vi "CF_Read_Config.vi"(4 "error in (no error)":errorcluster, 7 "Config Refnum":T1) -> (0 "error out":errorcluster, 2 "All Found?":bool, 3 "refnum out":T1)   [LabVIEW 2015]
uses:
  <vilib>/Utility/config.llb/Config Data RefNum.ctl
  <vilib>/Utility/config.llb/Read Key (Double).vi
  GSP_CF_Global.vi
  <vilib>/Utility/config.llb/NI_LVConfig.lvlib
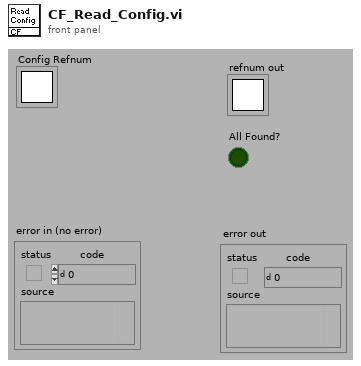
[diagram p1: front panel]
types:
  T1 = typedef "NI_LVConfig.lvlib/Config Data RefNum.ctl" = refnum<k1>
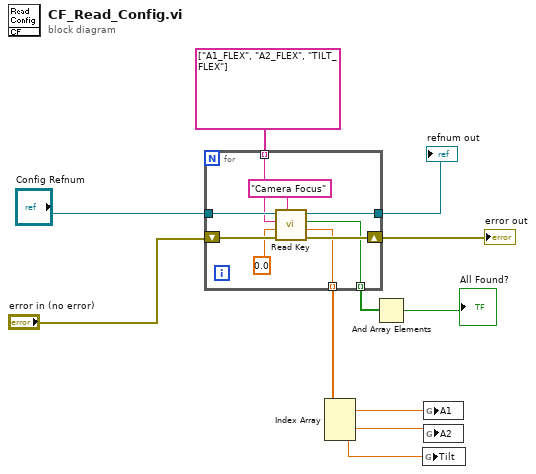
[diagram p0: block diagram]
diagram:
  n1 = for {
    tunnel: "Config Refnum" -> [w19]
    shift-right: [w17] -> w8
    shift-left: "error in (no error)" -> [w20]
    tunnel: [w16] -> w7
    tunnel: string[] ["A1_FLEX", "A2_FLEX", "TILT_FLEX"] -> [w15] mode=indexing
    tunnel: [w13] -> w5 mode=indexing
    tunnel: [w12] -> w6 mode=indexing
    n2 = call-poly <vilib>:"Read Key.vi"("section"="Camera Focus", "error in (no error)"=w20, "default value"=0.0, "key"=w15, "refnum"=w19) -> ("error out"=w17:errorcluster, "value"=w12:dbl, "found?"=w13:bool, "refnum out"=w16:T1)  [unwired: 3 in]
  }
  "error out" <- w8
  "refnum out" <- w7
  n3 = Index Array(array=w6) -> (element #1=w3:dbl, element #2=w2:dbl, element #3=w1:dbl)  [unwired: 3 in]
  n4 = And Array Elements(Boolean array=w5) -> (logical AND=→"All Found?":bool)
  n5 = global write "GSP_CF_Global.vi" "Tilt"(w1) -> ()
  n6 = global write "GSP_CF_Global.vi" "A1"(w3) -> ()
  n7 = global write "GSP_CF_Global.vi" "A2"(w2) -> ()
